vi "imageDrawGrid.vi"(0 "Image":T1, 1 "Image height":u32, 2 "Image width":u32) -> (7 "Image Out":T1)   [LabVIEW 2020]
uses:
  <vilib>/vision/Image Controls.llb/IMAQ Image.ctl
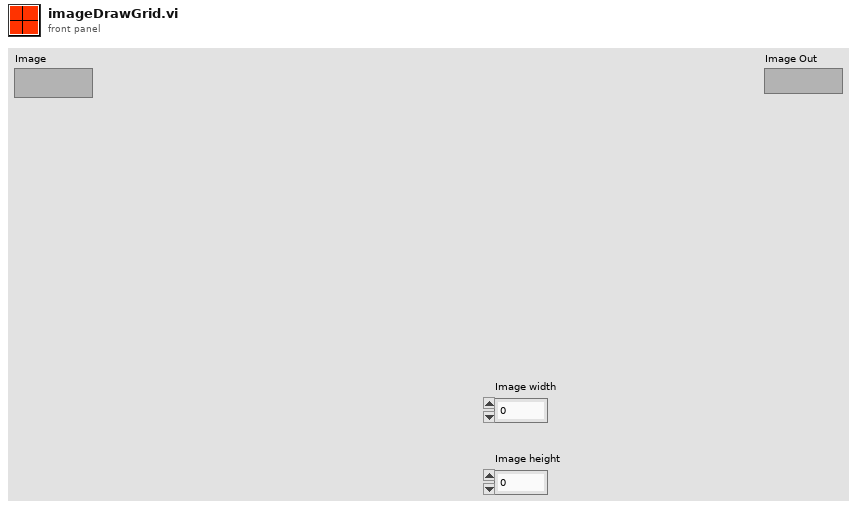
[diagram p1: front panel]
types:
  T1 = typedef "IMAQ Image.ctl" = refnum<image>
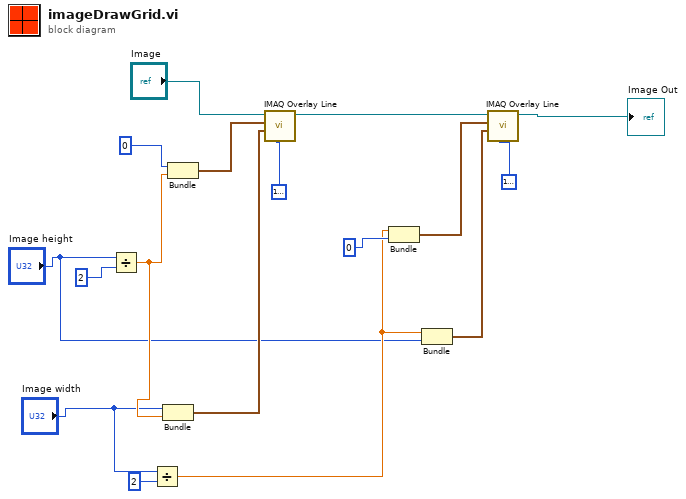
[diagram p0: block diagram]
diagram:
  n1 = Divide(x="Image height", y=u32 2) -> (x/y=w13:dbl)
  n2 = Divide(x="Image width", y=u32 2) -> (x/y=w4:dbl)
  n3 = Bundle("Image width"="Image width", w13) -> (w12:cluster{"Image width":u32, dbl})  [unwired: 1 in]
  n4 = Bundle(0, w13) -> (w14:cluster{i32, dbl})  [unwired: 1 in]
  n5 = call "IMAQ Overlay Line"("Color"=u32 16777222, "End Point"=w12, "Start Point"=w14, "Image"="Image") -> ("Image Out"=w10:T1)  [unwired: 6 in, 1 out]
  n6 = Bundle(w4, 0) -> (w5:cluster{dbl, i32})  [unwired: 1 in]
  n7 = Bundle(w4, "Image height"="Image height") -> (w2:cluster{dbl, "Image height":u32})  [unwired: 1 in]
  n8 = call "IMAQ Overlay Line"("Color"=u32 16777222, "End Point"=w2, "Start Point"=w5, "Image"=w10) -> ("Image Out"=→"Image Out":T1)  [unwired: 6 in, 1 out]
